vi "Autoscale_Channel.vi"(8 "error in":errorcluster, 10 "Channel":i32(ring)=1 items=["Channel 1"=1, "Channel 2"=2, "Channel 3"=3, "Channel 4"=4, "Function 1"=5, "Function 2"=6, "Function 3"=7, "Function 4"=8, "Memory 1"=9, "Memory 2"=10, "Memory 3"=11, "Memory 4"=12], 11 "VISA resource name":refnum<visa-resource-name>) -> (0 "error out":errorcluster, 3 "VISA resource name out":refnum<visa-resource-name>, 4 "Offset":dbl, 6 "VerticalRange":dbl)   [LabVIEW 2009]
uses:
  <instrlib>/Agilent 8000 Series/Agilent 8000 Series.lvlib
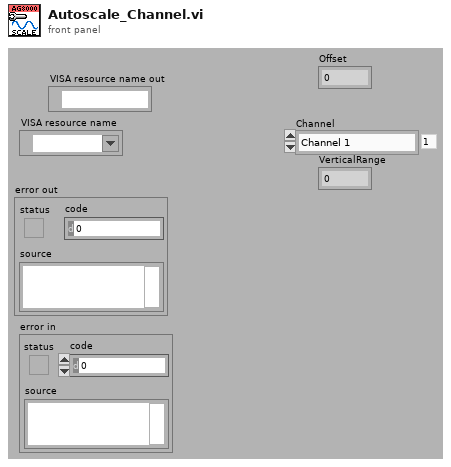
[diagram p1: front panel]
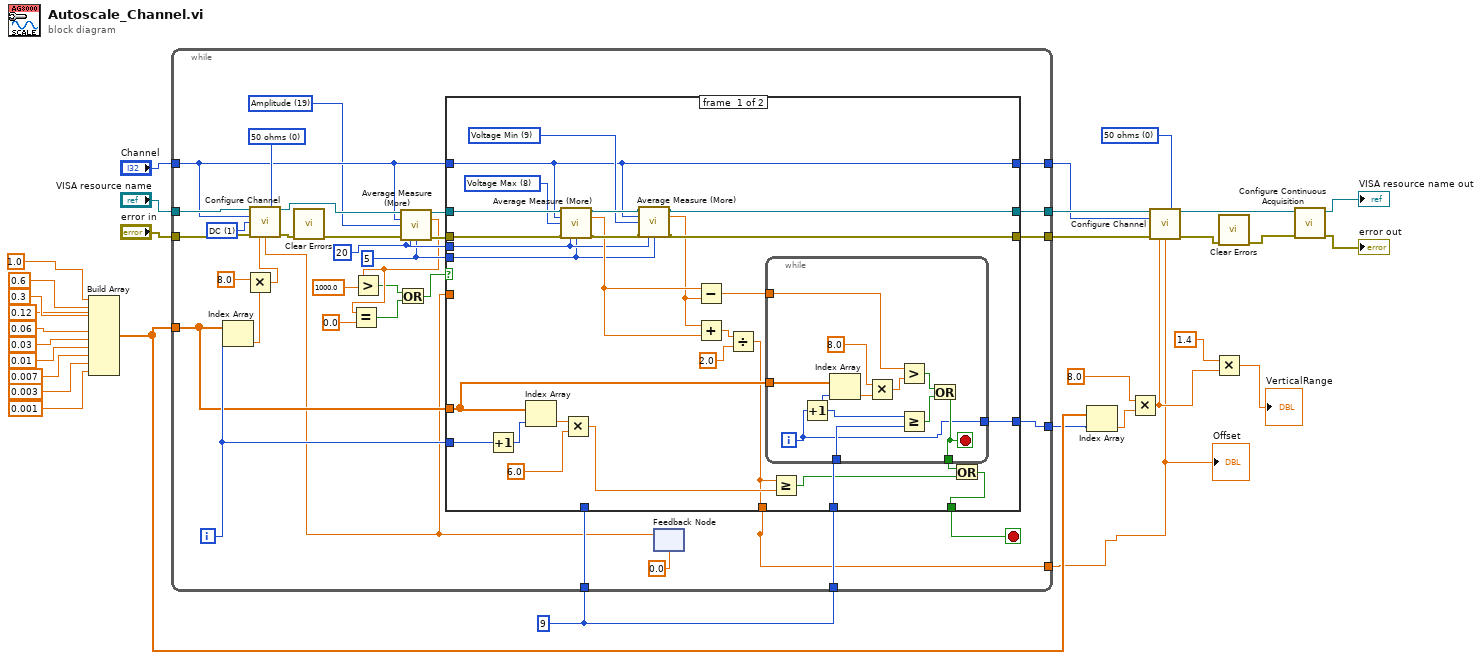
[diagram p0: block diagram]
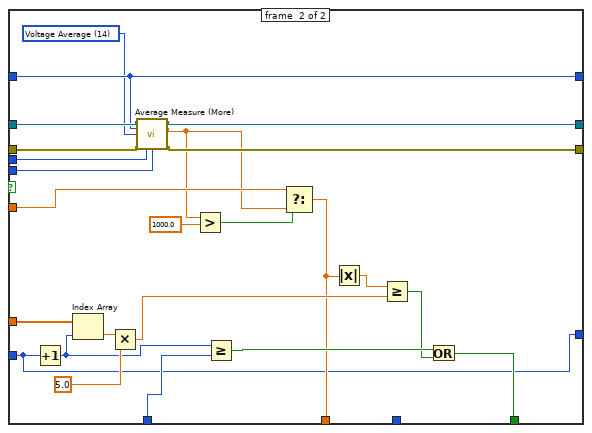
[diagram p2: hidden frame]
diagram:
  w16 = u32 0 items=["50 ohms", "1 Mohms"] ("Input Impedance (1: 1 Mohms)")
  w28 = 9 ("y")
  n1 = Build Array(1.0 ("element"), 0.6 ("element"), 0.3 ("element"), 0.12 ("element"), 0.06 ("element"), 0.03 ("element"), 0.01 ("element"), 0.007 ("element"), 0.003 ("element"), 0.001 ("element")) -> (w15:dbl[])
  n2 = while {
    tunnel: "Channel" -> [w39]
    tunnel: w28 -> [w60]
    tunnel: w28 -> [w58]
    tunnel: w15 -> [w51]
    tunnel: [w56] -> w19
    tunnel: [w55] -> w18
    tunnel: [w54] -> w17
    tunnel: "VISA resource name" -> [w53]
    tunnel: "error in" -> [w52]
    tunnel: [w49] -> w1
    tunnel: [w32] -> w7
    i -> [w57]
    stop <- w59 stop-if-true
    w40 = u32 5 ("Max Errors")
    w41 = u32 20 ("Averages")
    w47 = 1 items=["AC", "DC"] ("Vertical Coupling (1: DC)")
    w62 = u32 0 items=["50 ohms", "1 Mohms"] ("Input Impedance (1: 1 Mohms)")
    w38 = 19 items=["Rise Time", "Fall Time", "Frequency", "Period", "Voltage RMS(AC)", "Voltage RMS(DC)", "Voltage RMS (AC,cycle)", "Voltage RMS (DC,cycle)", "Voltage Max", "Voltage Min", "Voltage Middle", "Voltage Vpp", "Voltage High", "Voltage Low", "Voltage Average", "Voltage Average (cycle)", "Width Negative", "Width Positive", "Duty Cycle Positive", "Amplitude", "Overshoot", "Preshoot", "Voltage Base", "Voltage Upper", "Time Max", "Time Min", "Color Grade Crossing", "Color Grade Eye Width", "Color Grade Eye Height", "Color Grade Eye Q-Factory", "Color Grade Eye Duty Cycle Distortion(Percent)", "Color Grade Eye Duty Cycle Distortion(Time)", "Color Grade Eye Jitter(PP)", "Color Grade Eye Width(RMS)", "Cycle-cycle Duty Jitter(Rising)", "Cycle-cycle Duty Jitter(Falling)", "Cycle-cycle Jitter(Rising)", "Cycle-cycle Jitter(Falling)", "Cycle-cycle - Width", "Cycle-cycle + Width", "Date Rate", "Unit Interval", "FFT Delta Frequency", "FFT Delta Magnitude", "FFT Frequency", "FFT Magnitude", "Slew Rate", "Area (Entire Display)", "Area(Single Cycle)", "Duty Cycle (Rising)", "Duty Cycle (Falling)"] ("Measurement Function (0: Rise Time)")
    n3 = Index Array(array=w51, index=w57) -> (element=w64:dbl)
    n4 = Multiply(x=8.0 ("y"), y=w64) -> (x*y=w63:dbl)
    n5 = feedback #1(0.0 ("Measurement")) -> (w48:dbl)
    n6 = call <instrlib>:"Configure Channel.vi"("VISA resource name"=w53, "Input Impedance (1: 1 Mohms)"=w62, "Channel (1: Channel 1)"=w39, "Vertical Coupling (1: DC)"=w47, "error in (no error)"=w52, "Vertical Range (2.0 V)"=w63, "Vertical Offset (0.0 V)"=w48) -> ("VISA resource name out"=w45:refnum<visa-resource-name>, "error out"=w46:errorcluster)  [unwired: 7 in]
    n7 = call <vilib>:"Clear Errors.vi"("error in (no error)"=w46) -> ("error out"=w44:errorcluster)  [unwired: 6 in]
    n8 = call "Average Measure (More).vi"("VISA resource name"=w45, "Channel (1: Channel 1)"=w39, "Measurement Function (0: Rise Time)"=w38, "error in (no error)"=w44, "Averages"=w41, "Max Errors"=w40) -> ("VISA resource name out"=w42:refnum<visa-resource-name>, "Measure Average"=w36:dbl, "error out"=w43:errorcluster)  [unwired: 6 in, 1 out]
    n9 = Equal?(x=w36, y=0.0) -> (x = y?=w33:bool)
    n10 = Greater?(x=w36, y=1000.0) -> (0:w34:bool)
    n11 = Or(x=w34, y=w33) -> (x .or. y?=w35:bool)
    n12 = case shown="False" w35 {
      tunnel: w39 -> [w70 w109]
      tunnel: w43 -> [w74 w111]
      tunnel: w42 -> [w73 w110]
      tunnel: w60 -> [_ w126]
      tunnel: [w79 w120] -> w59
      tunnel: [w82 w119] -> w49
      tunnel: w58 -> [w91 _]
      tunnel: w51 -> [w85 w118]
      tunnel: w57 -> [w84 w115]
      tunnel: [w78 w113] -> w56
      tunnel: [w77 w112] -> w55
      tunnel: [w70 w109] -> w54
      tunnel: [w89 w115] -> w32
      tunnel: w48 -> [_ w114]
      tunnel: w41 -> [w67 w107]
      tunnel: w40 -> [w66 w106]
      frame #0 {
        w71 = 9 items=["Rise Time", "Fall Time", "Frequency", "Period", "Voltage RMS(AC)", "Voltage RMS(DC)", "Voltage RMS (AC,cycle)", "Voltage RMS (DC,cycle)", "Voltage Max", "Voltage Min", "Voltage Middle", "Voltage Vpp", "Voltage High", "Voltage Low", "Voltage Average", "Voltage Average (cycle)", "Width Negative", "Width Positive", "Duty Cycle Positive", "Amplitude", "Overshoot", "Preshoot", "Voltage Base", "Voltage Upper", "Time Max", "Time Min", "Color Grade Crossing", "Color Grade Eye Width", "Color Grade Eye Height", "Color Grade Eye Q-Factory", "Color Grade Eye Duty Cycle Distortion(Percent)", "Color Grade Eye Duty Cycle Distortion(Time)", "Color Grade Eye Jitter(PP)", "Color Grade Eye Width(RMS)", "Cycle-cycle Duty Jitter(Rising)", "Cycle-cycle Duty Jitter(Falling)", "Cycle-cycle Jitter(Rising)", "Cycle-cycle Jitter(Falling)", "Cycle-cycle - Width", "Cycle-cycle + Width", "Date Rate", "Unit Interval", "FFT Delta Frequency", "FFT Delta Magnitude", "FFT Frequency", "FFT Magnitude", "Slew Rate", "Area (Entire Display)", "Area(Single Cycle)", "Duty Cycle (Rising)", "Duty Cycle (Falling)"] ("Measurement Function (0: Rise Time)")
        w72 = 8 items=["Rise Time", "Fall Time", "Frequency", "Period", "Voltage RMS(AC)", "Voltage RMS(DC)", "Voltage RMS (AC,cycle)", "Voltage RMS (DC,cycle)", "Voltage Max", "Voltage Min", "Voltage Middle", "Voltage Vpp", "Voltage High", "Voltage Low", "Voltage Average", "Voltage Average (cycle)", "Width Negative", "Width Positive", "Duty Cycle Positive", "Amplitude", "Overshoot", "Preshoot", "Voltage Base", "Voltage Upper", "Time Max", "Time Min", "Color Grade Crossing", "Color Grade Eye Width", "Color Grade Eye Height", "Color Grade Eye Q-Factory", "Color Grade Eye Duty Cycle Distortion(Percent)", "Color Grade Eye Duty Cycle Distortion(Time)", "Color Grade Eye Jitter(PP)", "Color Grade Eye Width(RMS)", "Cycle-cycle Duty Jitter(Rising)", "Cycle-cycle Duty Jitter(Falling)", "Cycle-cycle Jitter(Rising)", "Cycle-cycle Jitter(Falling)", "Cycle-cycle - Width", "Cycle-cycle + Width", "Date Rate", "Unit Interval", "FFT Delta Frequency", "FFT Delta Magnitude", "FFT Frequency", "FFT Magnitude", "Slew Rate", "Area (Entire Display)", "Area(Single Cycle)", "Duty Cycle (Rising)", "Duty Cycle (Falling)"] ("Measurement Function (0: Rise Time)")
        n13 = Increment(x=w84) -> (x+1=w86:i32)
        n14 = Index Array(array=w85, index=w86) -> (element=w87:dbl)
        n15 = call "Average Measure (More).vi"("VISA resource name"=w73, "Channel (1: Channel 1)"=w70, "Measurement Function (0: Rise Time)"=w72, "error in (no error)"=w74, "Averages"=w67, "Max Errors"=w66) -> ("VISA resource name out"=w76:refnum<visa-resource-name>, "Measure Average"=w69:dbl, "error out"=w75:errorcluster)  [unwired: 6 in, 1 out]
        n16 = Multiply(x=w87, y=6.0) -> (x*y=w83:dbl)
        n17 = call "Average Measure (More).vi"("VISA resource name"=w76, "Channel (1: Channel 1)"=w70, "Measurement Function (0: Rise Time)"=w71, "error in (no error)"=w75, "Averages"=w67, "Max Errors"=w66) -> ("VISA resource name out"=w78:refnum<visa-resource-name>, "Measure Average"=w68:dbl, "error out"=w77:errorcluster)  [unwired: 6 in, 1 out]
        n18 = Subtract(x=w69, y=w68) -> (x-y=w90:dbl)
        n19 = Add(x=w68, y=w69) -> (x+y=w92:dbl)
        n20 = Divide(x=w92, y=2.0) -> (x/y=w82:dbl)
        n21 = while {
          tunnel: w91 -> [w104]
          tunnel: w85 -> [w103]
          tunnel: w90 -> [w99]
          tunnel: [w96] -> w81
          tunnel: [w95] -> w89
          i -> [w95]
          stop <- w96 stop-if-true
          n22 = Increment(x=w95) -> (x+1=w94:i32)
          n23 = Index Array(array=w103, index=w94) -> (element=w102:dbl)
          n24 = Multiply(x=8.0, y=w102) -> (x*y=w100:dbl)
          n25 = Greater?(x=w99, y=w100) -> (0:w98:bool)
          n26 = Greater Or Equal?(x=w94, y=w104) -> (x >= y?=w97:bool)
          n27 = Or(x=w98, y=w97) -> (x .or. y?=w96:bool)
        }
        n28 = Greater Or Equal?(x=w82, y=w83) -> (x >= y?=w80:bool)
        n29 = Or(x=w81, y=w80) -> (x .or. y?=w79:bool)
      }
      frame #1 {
        w108 = 14 items=["Rise Time", "Fall Time", "Frequency", "Period", "Voltage RMS(AC)", "Voltage RMS(DC)", "Voltage RMS (AC,cycle)", "Voltage RMS (DC,cycle)", "Voltage Max", "Voltage Min", "Voltage Middle", "Voltage Vpp", "Voltage High", "Voltage Low", "Voltage Average", "Voltage Average (cycle)", "Width Negative", "Width Positive", "Duty Cycle Positive", "Amplitude", "Overshoot", "Preshoot", "Voltage Base", "Voltage Upper", "Time Max", "Time Min", "Color Grade Crossing", "Color Grade Eye Width", "Color Grade Eye Height", "Color Grade Eye Q-Factory", "Color Grade Eye Duty Cycle Distortion(Percent)", "Color Grade Eye Duty Cycle Distortion(Time)", "Color Grade Eye Jitter(PP)", "Color Grade Eye Width(RMS)", "Cycle-cycle Duty Jitter(Rising)", "Cycle-cycle Duty Jitter(Falling)", "Cycle-cycle Jitter(Rising)", "Cycle-cycle Jitter(Falling)", "Cycle-cycle - Width", "Cycle-cycle + Width", "Date Rate", "Unit Interval", "FFT Delta Frequency", "FFT Delta Magnitude", "FFT Frequency", "FFT Magnitude", "Slew Rate", "Area (Entire Display)", "Area(Single Cycle)", "Duty Cycle (Rising)", "Duty Cycle (Falling)"] ("Measurement Function (0: Rise Time)")
        n30 = Increment(x=w115) -> (x+1=w116:i32)
        n31 = Index Array(array=w118, index=w116) -> (element=w117:dbl)
        n32 = Multiply(x=w117, y=5.0) -> (x*y=w124:dbl)
        n33 = call "Average Measure (More).vi"("VISA resource name"=w110, "Channel (1: Channel 1)"=w109, "Measurement Function (0: Rise Time)"=w108, "error in (no error)"=w111, "Averages"=w107, "Max Errors"=w106) -> ("VISA resource name out"=w113:refnum<visa-resource-name>, "Measure Average"=w105:dbl, "error out"=w112:errorcluster)  [unwired: 6 in, 1 out]
        n34 = Greater?(x=w105, y=1000.0) -> (0:w127:bool)
        n35 = Greater Or Equal?(x=w116, y=w126) -> (x >= y?=w122:bool)
        n36 = Select(t=w114, s=w127, f=w105) -> (s? t:f=w119:dbl)
        n37 = Absolute Value(x=w119) -> (abs(x)=w123:dbl)
        n38 = Greater Or Equal?(x=w123, y=w124) -> (x >= y?=w121:bool)
        n39 = Or(x=w122, y=w121) -> (x .or. y?=w120:bool)
      }
    }
  }
  "Offset" <- w1
  n40 = Index Array(array=w15, index=w7) -> (element=w10:dbl)
  n41 = Multiply(x=8.0, y=w10) -> (x*y=w4:dbl)
  n42 = call <instrlib>:"Configure Channel.vi"("VISA resource name"=w19, "Input Impedance (1: 1 Mohms)"=w16, "Channel (1: Channel 1)"=w17, "error in (no error)"=w18, "Vertical Range (2.0 V)"=w4, "Vertical Offset (0.0 V)"=w1) -> ("VISA resource name out"=w14:refnum<visa-resource-name>, "error out"=w8:errorcluster)  [unwired: 8 in]
  n43 = Multiply(x=1.4, y=w4) -> (x*y=→"VerticalRange":dbl)
  n44 = call <vilib>:"Clear Errors.vi"("error in (no error)"=w8) -> ("error out"=w9:errorcluster)  [unwired: 6 in]
  n45 = call <instrlib>:"Configure Continuous Acquisition.vi"("error in (no error)"=w9, "VISA resource name"=w14) -> ("error out"=→"error out":errorcluster, "VISA resource name out"=→"VISA resource name out":refnum<visa-resource-name>)  [unwired: 8 in]
